vi "Keithley 2450 Read Multiple R.vi"(6 "num exclude":u32=4, 7 "Num Meas":u32=10, 8 "Compliance  Level (0.1)":dbl=0.1, 9 "Output Level (0)":dbl, 10 "Source Mode  (0: Voltage)":u16(ring) items=["Voltage", "Current"], 11 "VISA resource name":refnum<visa-resource-name>) -> (0 "Resistance":sgl[](array[numeric]))   [LabVIEW 2024]
doc: "This example shows how to configure a measurement and take multiple readings."
uses:
  Keithley/Keithley 2450/Keithley 2450.lvlib
  Keithley/archive/Keithley 24XX/Keithley 24XX.lvlib
panel:
  out "error out":errorcluster
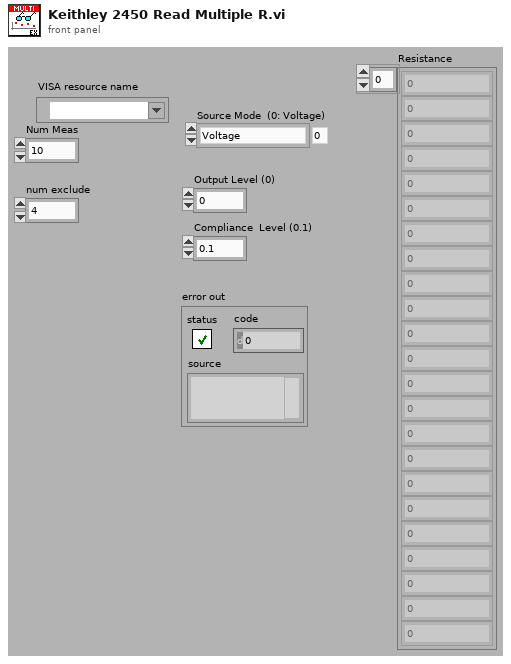
[diagram p1: front panel]
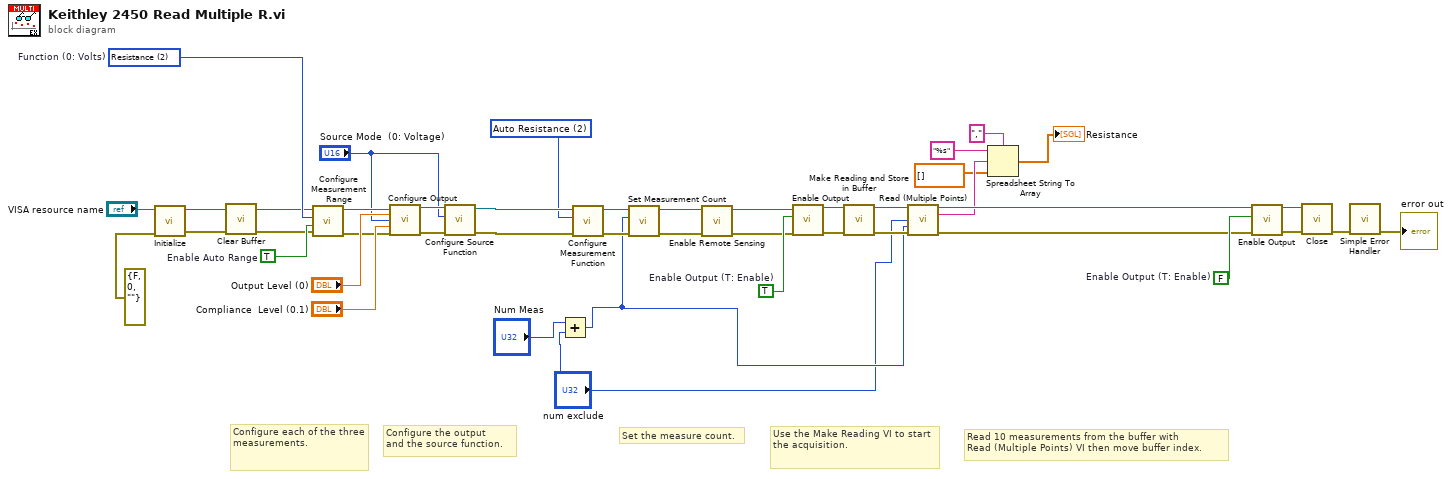
[diagram p0: block diagram]
diagram:
  w4 = u16 2 items=["Volts", "Current", "Auto Resistance", "Manual Resistance", "Digitize Voltage", "Digitize Current"] ("Function (0: Volts)")
  w15 = TRUE  # Enable Output (T: Enable)
  w37 = FALSE  # Enable Output (T: Enable)
  w42 = u16 2 items=["Volts", "Current", "Resistance"]  # Function (0: Volts)
  w25 = TRUE  # Enable Auto Range
  # "Read 10 measurements from the buffer with \nRead (Multiple Points) VI then move buffer index."
  # "Set the measure count."
  # "Use the Make Reading VI to start the acquisition."
  # "Configure the output \nand the source function."
  # "Configure each of the three measurements."
  n1 = call "Initialize.vi"("error in (no error)"=errorcluster {"status"=FALSE, "code"=0, "source"=""}, "VISA resource name"="VISA resource name") -> ("error out"=w7:errorcluster, "VISA resource name out"=w8:refnum<visa-resource-name>)  [unwired: 8 in]
  n2 = call "Clear Buffer.vi"("VISA resource name"=w8, "error in (no error)"=w7) -> ("VISA resource name out"=w5:refnum<visa-resource-name>, "error out"=w6:errorcluster)  [unwired: 12 in]
  n3 = call "Configure Measurement Range.vi"("error in (no error)"=w6, "Enable Auto Range (T:Enable)"=w25, "Function (0: Volts)"=w42, "VISA resource name"=w5) -> ("error out"=w35:errorcluster, "VISA resource name out"=w36:refnum<visa-resource-name>)  [unwired: 6 in]
  n4 = call "Configure Output.vi"("VISA resource name"=w36, "Source Level (0)"="Output Level (0)", "Source Mode  (0: Voltage)"="Source Mode  (0: Voltage)", "Source Limit Level (0.1)"="Compliance  Level (0.1)", "error in (no error)"=w35) -> ("VISA resource name out"=w31:refnum<visa-resource-name>, "error out"=w32:errorcluster)  [unwired: 9 in]
  n5 = call "Configure Source Function.vi"("error in (no error)"=w32, "Function (0: Volts)"="Source Mode  (0: Voltage)", "VISA resource name"=w31) -> ("error out"=w29:errorcluster, "VISA resource name out"=w30:refnum<visa-resource-name>)  [unwired: 7 in]
  n6 = Add(x="Num Meas", y="num exclude") -> (x+y=w3:u32)
  n7 = call "Configure Measurement Function.vi"("error in (no error)"=w29, "Function (0: Volts)"=w4, "VISA resource name"=w30) -> ("error out"=w24:errorcluster, "VISA resource name out"=w23:refnum<visa-resource-name>)  [unwired: 7 in]
  n8 = call "Set Measurement Count.vi"("error in (no error)"=w24, "Measurement Count"=w3, "VISA resource name"=w23) -> ("error out"=w10:errorcluster, "VISA resource name out"=w12:refnum<visa-resource-name>)  [unwired: 7 in]
  n9 = call "Enable Remote Sensing.vi"("error in (no error)"=w10, "VISA resource name"=w12) -> ("error out"=w9:errorcluster, "VISA resource name out"=w11:refnum<visa-resource-name>)  [unwired: 8 in]
  n10 = call "Enable Output.vi"("error in (no error)"=w9, "Enable Output (T: Enable)"=w15, "VISA resource name"=w11) -> ("error out"=w13:errorcluster, "VISA resource name out"=w14:refnum<visa-resource-name>)  [unwired: 7 in]
  n11 = call "Make Reading and Store in Buffer.vi"("VISA resource name"=w14, "error in (no error)"=w13) -> ("VISA resource name out"=w17:refnum<visa-resource-name>, "error out"=w16:errorcluster)  [unwired: 12 in]
  n12 = call "Read (Multiple Points).vi"("VISA resource name"=w17, "Start Index (1)"="num exclude", "End Index (1)"=w3, "error in (no error)"=w16) -> ("VISA resource name out"=w34:refnum<visa-resource-name>, "Data out"=w22:string, "error out"=w33:errorcluster)  [unwired: 9 in]
  n13 = Spreadsheet String To Array(delimiter (Tab)=",", format string="%s", spreadsheet string=w22, array type (2D Dbl)=dbl[] []) -> (array=→"Resistance":dbl[])
  n14 = call "Enable Output.vi"("error in (no error)"=w33, "Enable Output (T: Enable)"=w37, "VISA resource name"=w34) -> ("error out"=w38:errorcluster, "VISA resource name out"=w39:refnum<visa-resource-name>)  [unwired: 7 in]
  n15 = call "Close.vi"("error in (no error)"=w38, "VISA resource name"=w39) -> ("error out"=w44:errorcluster)  [unwired: 9 in]
  n16 = call <vilib>:"Simple Error Handler.vi"("error in (no error)"=w44) -> ("error out"=→"error out":errorcluster)  [unwired: 4 in, 4 out]
